vi "Write Calibrate.vi"(8 "error in (no error)":errorcluster, 10 "Calibrate?":refnum<notifier>, 11 "Pcal GUI in":refnum<class "Pcal GUI.lvclass">) -> (0 "error out":errorcluster, 3 "Pcal GUI out":refnum<class "Pcal GUI.lvclass">)   [LabVIEW 2015, in "Pcal GUI.lvclass"]
uses:
  Pcal GUI.lvclass
  Pcal GUI.lvclass/Pcal GUI.ctl
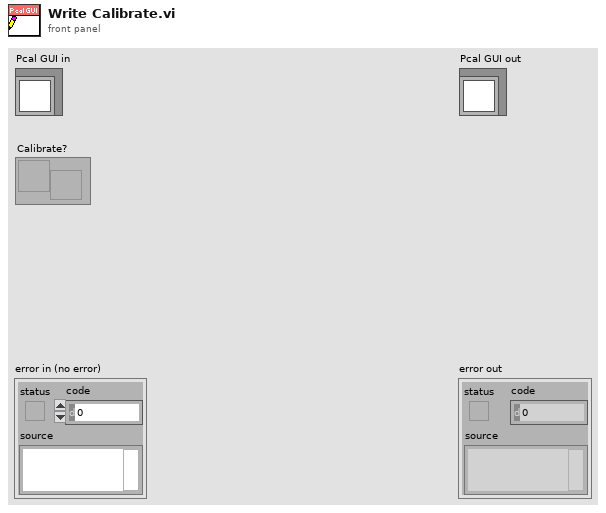
[diagram p1: front panel]
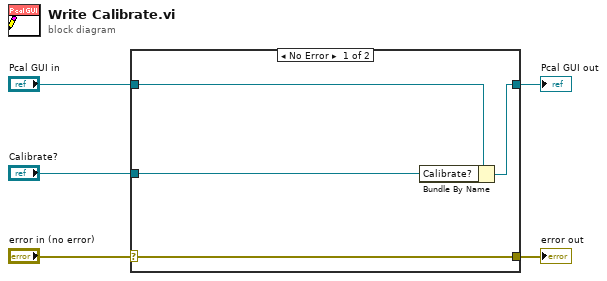
[diagram p0: block diagram]
diagram:
  n1 = case shown="No Error" "error in (no error)" {
    selector: "error in (no error)" -> [w9 w10]
    tunnel: [w9 w10] -> w4
    tunnel: [w7 w11] -> w2
    tunnel: "Pcal GUI in" -> [w8 w11]
    tunnel: "Calibrate?" -> [w6 _]
    frame No Error {
      n2 = Bundle By Name(cluster=w8, "Calibrate?"=w6) -> (w7:refnum<class "Pcal GUI.lvclass">)
    }
    frame Error {
    }
  }
  "error out" <- w4
  "Pcal GUI out" <- w2
